vi "Config_Distancias_Sistema.vi"() -> ()   [LabVIEW 2015]
uses:
  <vilib>/Utility/file.llb/Write Delimited Spreadsheet (string).vi
panel:
  out "new file path (Not A Path if cancelled)":path
  in  "Tab Control":enum32{"Distancias", "Valores"}(tab)
  in  "Número de máximo de\nunidades por convoy":i16=2
  in  "Ruta donde se guarda el archivo configuracion.txr":path=path "configuracion.txt"
  in  "Inductivo":dbl=15.0
  in  "Distancia entre ejes":dbl=2.2
  in  "X3":dbl=5.44
  in  "X2":dbl=12.5
  in  "X1":dbl=2.9
  in  "Acelerómetro 4":dbl=8.51
  in  "Acelerómetro 3":dbl=6.51
  in  "Acelerómetro 2":dbl=4.51
  in  "Acelerómetro 1":dbl=2.51
  in  "Número de coches\npor unidad":i16=4
  in  "Compensación de distancia del frontal":dbl
  in  "Ventana":dbl=2.72
  out "Distancia entre ejes":dbl[](array[numeric])
  out "F-format string":string[](array[string])
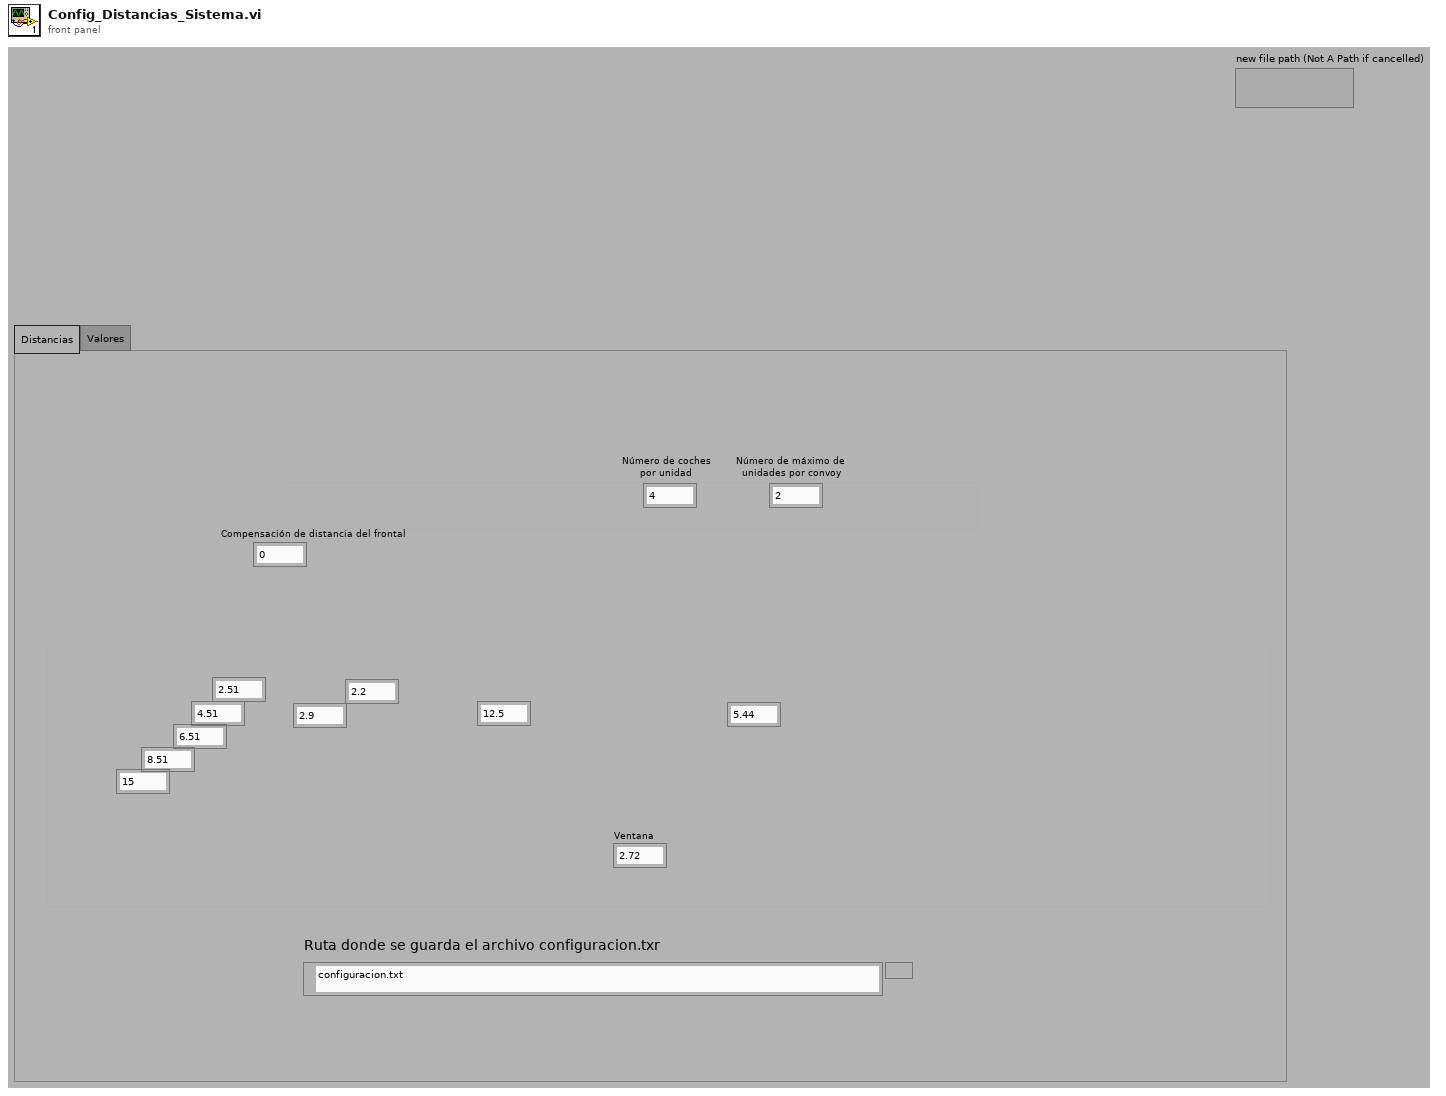
[diagram p1: front panel]
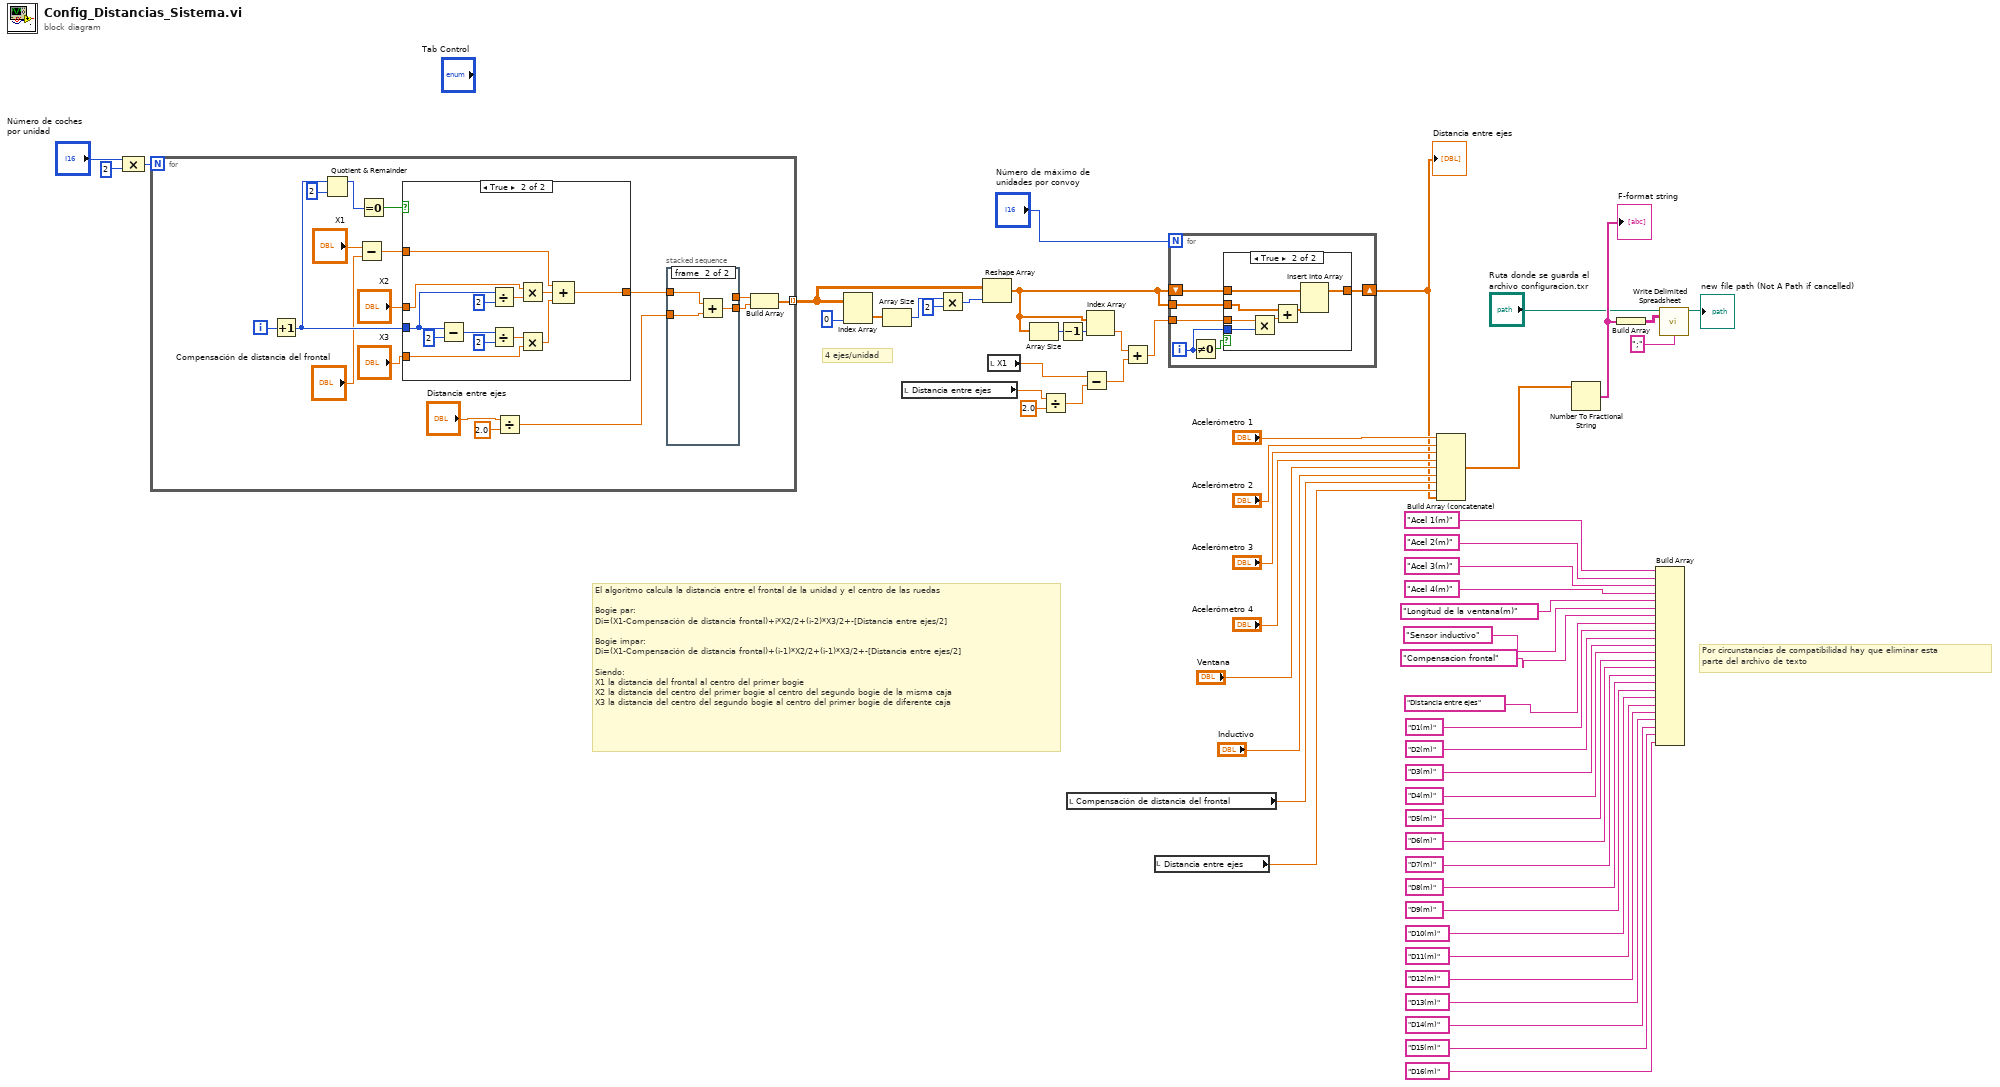
[diagram p0: block diagram]
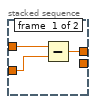
[diagram p3: hidden frame]
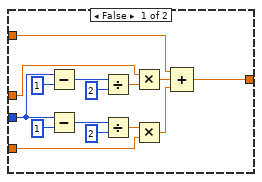
[diagram p4: hidden frame]
diagram:
  # "4 ejes/unidad"
  # "Por circunstancias de compatibilidad hay que eliminar esta\nparte del archivo de texto"
  # "El algoritmo calcula la distancia entre el frontal de la unidad y el centro de las ruedas\n\nBogie par:\nDi=(X1-Compensación de distancia frontal)+i*X2/2+(i-2)*X3/2+-[Distancia entre ejes/2]\n\nBogie impar:\nDi=(X1-Compensación de distancia frontal)+(i-1)*X2/2+(i-1)*X3/2+-[Distancia entre ejes/2]      \n\nSiendo:\nX1 la distancia del frontal al centro del primer bogie\nX2 la distancia del centro del primer bogie al centro del segundo bogie de la misma caja\nX3 la distancia del centro del segundo bogie al centro del primer bogie de diferente caja"
  n1 = Compound Arithmetic op=MULTIPLY("Número de coches\npor unidad", i16 2 ("y")) -> (w12:i16)
  n2 = for {
    N: w12 -> [_]
    tunnel: [w68] -> w59 mode=indexing
    i -> [w76]
    n3 = Increment(x=w76) -> (x+1=w72:i32)
    n4 = Quotient & Remainder(x=w72, y=2) -> (x-y*floor(x/y)=w74:i32)  [unwired: 1 out]
    n5 = Subtract(x="X1", y="Compensación de distancia del frontal") -> (x-y=w66:dbl)
    n6 = Equal To 0?(x=w74) -> (x = 0?=w73:bool)
    n7 = case shown="True" w73 {
      tunnel: w72 -> [w88 w108]
      tunnel: [w86 w101] -> w71
      tunnel: "X3" -> [w83 w100]
      tunnel: "X2" -> [w84 w99]
      tunnel: w66 -> [w85 w98]
      frame False {
        n8 = Subtract(x=w88, y=1) -> (x-y=w87:i32)
        n9 = Subtract(x=w88, y=1) -> (x-y=w91:i32)
        n10 = Divide(x=w87, y=2) -> (x/y=w94:dbl)
        n11 = Divide(x=w91, y=2) -> (x/y=w95:dbl)
        n12 = Multiply(x=w84, y=w94) -> (x*y=w96:dbl)
        n13 = Multiply(x=w95, y=w83) -> (x*y=w97:dbl)
        n14 = Compound Arithmetic op=ADD(w85, w96, w97) -> (w86:dbl)
      }
      frame True {
        n15 = Subtract(x=w108, y=2) -> (x-y=w109:i32)
        n16 = Divide(x=w108, y=2) -> (x/y=w105:dbl)
        n17 = Divide(x=w109, y=2) -> (x/y=w104:dbl)
        n18 = Multiply(x=w99, y=w105) -> (x*y=w103:dbl)
        n19 = Multiply(x=w104, y=w100) -> (x*y=w102:dbl)
        n20 = Compound Arithmetic op=ADD(w98, w103, w102) -> (w101:dbl)
      }
    }
    n21 = Divide(x="Distancia entre ejes", y=2.0) -> (x/y=w60:dbl)
    n22 = stacked-sequence {
      tunnel: w71 -> [w79 w82]
      tunnel: [w78 _] -> w70
      tunnel: [_ w81] -> w69
      tunnel: w60 -> [w77 w80]
      frame #0 {
        n23 = Subtract(x=w79, y=w77) -> (x-y=w78:dbl)
      }
      frame #1 {
        n24 = Add(x=w82, y=w80) -> (x+y=w81:dbl)
      }
    }
    n25 = Build Array(w70, w69) -> (w68:dbl[])
  }
  n26 = Index Array(array=w59, index (col)=0 ("disabled index (col)")) -> (element=w57:dbl[])  [unwired: 1 in]
  n27 = Array Size(array=w57) -> (size(s)=w56:i32)
  n28 = local read "Distancia entre ejes"() -> (w8:dbl)
  n29 = Multiply(x=w56, y=2) -> (x*y=w54:i32)
  n30 = Reshape Array(w59, w54) -> (w2:dbl[])
  n31 = local read "X1"() -> (w11:dbl)
  n32 = Array Size(array=w2) -> (size(s)=w6:i32)
  n33 = Divide(x=w8, y=2.0) -> (x/y=w7:dbl)
  n34 = Decrement(x=w6) -> (x-1=w5:i32)
  n35 = local read "Compensación de distancia del frontal"() -> (w22:dbl)
  n36 = Subtract(x=w11, y=w7) -> (x-y=w3:dbl)
  n37 = Index Array(array=w2, index=w5) -> (element=w4:dbl)
  n38 = Add(x=w4, y=w3) -> (x+y=w1:dbl)
  n39 = local read "Distancia entre ejes"() -> (w20:dbl)
  n40 = for {
    N: "Número de máximo de\nunidades por convoy" -> [_]
    shift-right: [w115] -> w15
    shift-left: w2 -> [w114]
    tunnel: w2 -> [w113]
    tunnel: w1 -> [w111]
    i -> [w112]
    n41 = Not Equal To 0?(x=w112) -> (x != 0?=w116:bool)
    n42 = case shown="True" w116 {
      tunnel: w114 -> [w117 w123]
      tunnel: [w117 w124] -> w115
      tunnel: w113 -> [_ w119]
      tunnel: w112 -> [_ w122]
      tunnel: w111 -> [_ w121]
      frame False {
      }
      frame True {
        n43 = Multiply(x=w121, y=w122) -> (x*y=w120:dbl)
        n44 = Add(x=w119, y=w120) -> (x+y=w118:dbl[])
        n45 = Insert Into Array(array=w123, new element=w118) -> (w124:dbl[])  [unwired: 1 in]
      }
    }
  }
  "Distancia entre ejes" <- w15
  n46 = Build Array (concatenate)("Acelerómetro 1", "Acelerómetro 2", "Acelerómetro 3", "Acelerómetro 4", "Ventana", "Inductivo", w22, w20, w15) -> (w27:dbl[])
  n47 = Number To Fractional String(number=w27) -> (F-format string=w25:string[])  [unwired: 3 out]
  "F-format string" <- w25
  n48 = Build Array(w25) -> (w17:string[][])
  n49 = Build Array("Acel 1(m)", "Acel 2(m)", "Acel 3(m)", "Acel 4(m)", "Longitud de la ventana(m)", "Sensor inductivo", "Compensacion frontal", "Distancia entre ejes", "D1(m)", "D2(m)", "D3(m)", "D4(m)", "D5(m)", "D6(m)", "D7(m)", "D8(m)", "D9(m)", "D10(m)", "D11(m)", "D12(m)", "D13(m)", "D14(m)", "D15(m)", "D16(m)") -> ()  [unwired: 1 out]
  n50 = call-poly <vilib>:"Write Delimited Spreadsheet.vi"("file path (dialog if empty)"="Ruta donde se guarda el archivo configuracion.txr", "2D data"=w17, "delimiter (\\t)"=";" ("delimiter (\\t)")) -> ("new file path (Not A Path if cancelled)"=→"new file path (Not A Path if cancelled)":path)  [unwired: 11 in, 1 out]
